vi "6.单周期循环.vi"() -> ()   [LabVIEW 2019]
uses:
  <vilib>/Platform/TimedLoop/XDataNode/timing_clust.ctl
  <vilib>/Platform/TimedLoop/XDataNode/nitl_modes.ctl
  <vilib>/Platform/TimedLoop/XDataNode/wakeup.ctl
  <vilib>/rvi/Emulation/niFpgaSctlEmulationGetInTimedLoop.vi
  <vilib>/rvi/Emulation/niFpgaEmulationReportErrorSimple.vi
  <vilib>/rvi/Emulation/niFpgaGetClockAttributes.vi
  <vilib>/rvi/Emulation/niFpgaCriticalErrorInLSC.vi
  <vilib>/rvi/eio/common/nirviEmuTemplateMethod_errors.vi
  <vilib>/Platform/TimedLoop/XDataNode/XDataNode.xnode
  <vilib>/eio/EIONode/EIONode.xnode
  <vilib>/Platform/TimedLoop/XDataNode/XDNodeRunTimeDep.lvlib
panel:
  out "Counters":u8
  out "循环时间":u32
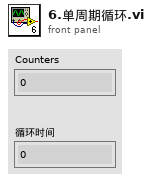
[diagram p1: front panel]
types:
  T1 = typedef "XDNodeRunTimeDep.lvlib/timing_clust.ctl" = cluster{"Expected End [f-1]":u64, "Actual End [f-1]":u64, "Finished Late? [f-1]":bool, "Expected End [i-1]":u64, "Actual End [i-1]":u64, "Finished Late? [i-1]":bool, "Expected Start [i]":u64, "Actual Start [i]":u64, "Expected Start [f]":u64, "Actual Start [f]":u64, "Source Name":string, "Structure Name":string, "Period":i64, "Deadline":i64, "Offset":i64, "Start":i64, "Priority":i32, "Timeout":i32, "Mode":T2, "Wakeup Reason":T3, "Error":errorcluster, "Source Type":string, "Secondary Source Type":string, "Global End Time":u64, "Global Start Time":u64, "Frame Duration":u64, "Iteration Duration":u64, "Assigned CPU":i32, "I/O Scan Engine Mode":u32}
  T2 = typedef "XDNodeRunTimeDep.lvlib/nitl_modes.ctl" = enum32{"No Change", "Process missed periods, maintain original phase", "Discard missed periods, maintain original phase", "Process missed periods, ignore original phase", "Discard missed periods, ignore original phase"}
  T3 = typedef "XDNodeRunTimeDep.lvlib/wakeup.ctl" = enum32{"Normal", "Aborted", "Asynchronous wakeup", "Timing source error", "Timed loop error", "Timeout"}
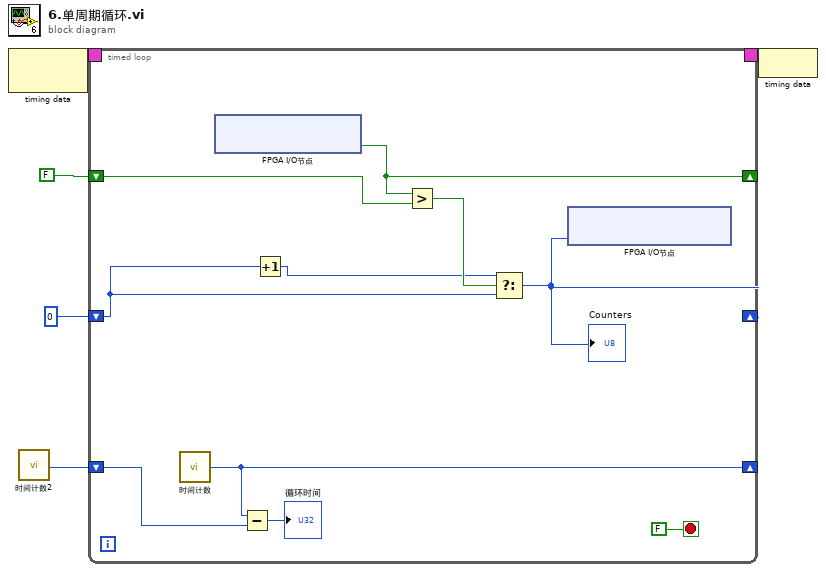
[diagram p0: block diagram]
diagram:
  n1 = node-c288() -> (w2:T1)  [unwired: 1 in]
  n2 = call "时间计数2"() -> ("Tick Count(Ticks)"=w3:u32)
  n3 = timed-loop {
    shift-right: [w13] -> _
    shift-left: FALSE -> [w14]
    shift-right: [w9] -> _
    shift-left: u8 0 -> [w10]
    shift-right: [w8] -> _
    shift-left: w3 -> [w7]
    timing: w2 -> [_]
    timing-out: [_] -> w1
    stop <- FALSE stop-if-true
    n4 = call "时间计数"() -> ("Tick Count(Ticks)"=w8:u32)
    n5 = xnode "FPGA I/O节点"() -> ("ConnectorA/DIO1"=w13:bool)  [unwired: 1 in, 1 out]
    n6 = Subtract(x=w8, y=w7) -> (x-y=→"循环时间":u32)
    n7 = Increment(x=w10) -> (x+1=w11:u8)
    n8 = Greater?(x=w13, y=w14) -> (0:w12:bool)
    n9 = Select(t=w11, s=w12, f=w10) -> (s? t:f=w9:u8)
    "Counters" <- w9
    n10 = xnode "FPGA I/O节点"("ConnectorA/DIO15:8"=w9) -> ()  [unwired: 1 in, 1 out]
  }
  n11 = node-c288(w1) -> ()
